vi "Fill in inside.vi"(9 "Starting Node":T1={"Row"=1, "Column"=1}, 11 "Array in":bool[][](array[boolean])) -> (3 "Array out":bool[][](array[boolean]))   [LabVIEW 2023]
uses:
  Problem-18/Cluster_Point.ctl
panel:
  out "ITTERATIONS":i32
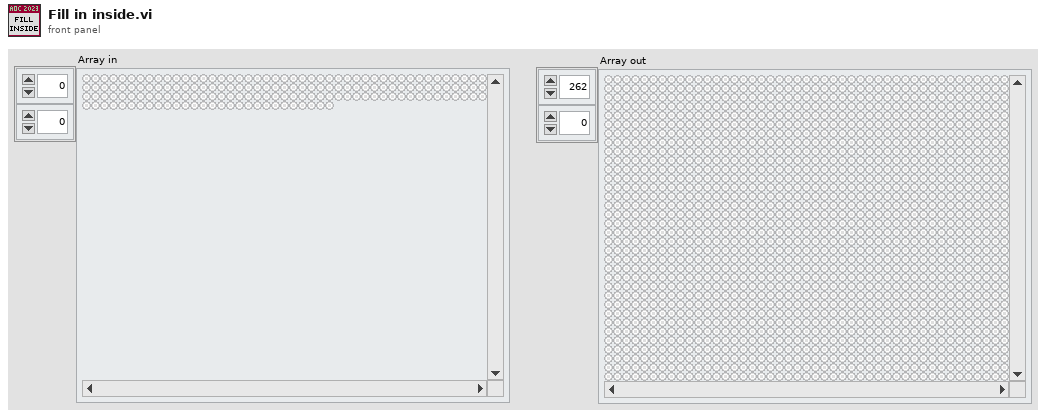
[diagram p1: front panel]
types:
  T1 = typedef "Cluster_Point.ctl" = cluster{"Row":i32, "Column":i32}
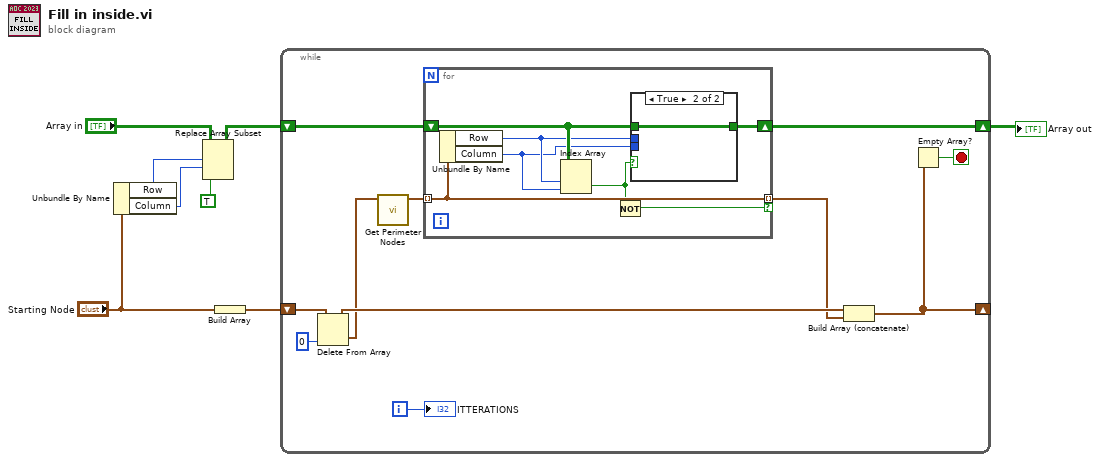
[diagram p0: block diagram]
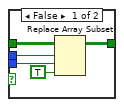
[diagram p2: hidden frame]
diagram:
  n1 = Unbundle By Name("Starting Node") -> ("Row"=w6:i32, "Column"=w5:i32)
  n2 = Replace Array Subset(array="Array in", new element=TRUE ("new element/subarray"), index (row)=w6, index (col)=w5) -> (w7:bool[][])
  n3 = Build Array("Starting Node") -> (w2:T1[])
  n4 = while {
    shift-right: [w12] -> w1
    shift-left: w7 -> [w13]
    shift-right: [w11] -> _
    shift-left: w2 -> [w19]
    i -> [w9]
    stop <- w16 stop-if-true
    n5 = Delete From Array(array=w19, index=0) -> (deleted portion=w15:T1, array with subset deleted=w17:T1[])  [unwired: 1 in]
    n6 = call "Get Perimeter Nodes.vi"("Point"=w15) -> ("Array"=w14:T1[])  [unwired: 10 in]
    n7 = for {
      tunnel: w14 -> [w26] mode=indexing
      shift-right: [w21] -> w12
      shift-left: w13 -> [w24]
      tunnel: [w26] -> w10 mode=indexing if=w25
      n8 = Unbundle By Name(w26) -> ("Row"=w23:i32, "Column"=w22:i32)
      n9 = Index Array(array=w24, index (row)=w23, index (col)=w22) -> (element=w20:bool)
      n10 = Not(x=w20) -> (.not. x?=w25:bool)
      n11 = case shown="True" w20 {
        tunnel: w24 -> [w31 w32]
        tunnel: w23 -> [w30 _]
        tunnel: w22 -> [w29 _]
        tunnel: [w27 w32] -> w21
        frame False {
          n12 = Replace Array Subset(array=w31, new element=TRUE ("new element/subarray"), index (row)=w30, index (col)=w29) -> (w27:bool[][])
        }
        frame True {
        }
      }
    }
    n13 = Build Array (concatenate)(w17, w10) -> (w11:T1[])
    n14 = Empty Array?(array=w11) -> (empty?=w16:bool)
    "ITTERATIONS" <- w9
  }
  "Array out" <- w1
